vi "AlliGator Settings Event Refnum.vi"(1 "AlliGator Settings Event":T1, 3 "Error In":errorcluster) -> (7 "AlliGator Settings Event Refnum":refnum<user-event>, 9 "Error Out":errorcluster)   [LabVIEW 2021, in "AlliGator Settings.lvlib"]
doc: "Sends user event to the Settings window."
uses:
  AlliGator Settings.lvlib
  AlliGator Settings Event.ctl
  AlliGator Settings Window Messages.ctl
panel:
  # "see the AlliGator License on the block diagram (Ctrl+E or Window:Show Block Diagram)"
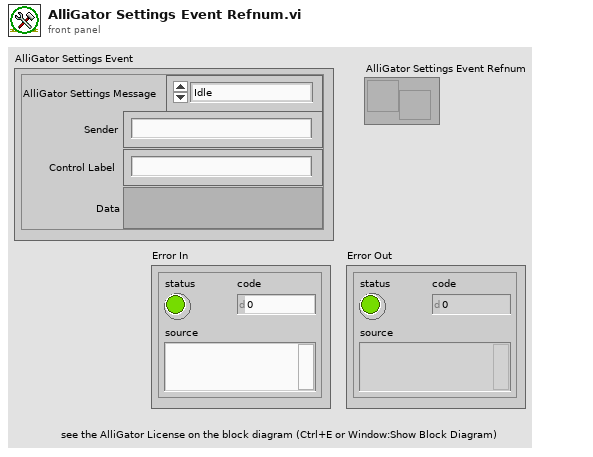
[diagram p1: front panel]
types:
  T1 = typedef "AlliGator Settings.lvlib/AlliGator Settings Event.ctl" = cluster{"AlliGator Settings Message":T2, "Sender":string, "Control Label":string, "Data":variant}
  T2 = typedef "AlliGator Settings.lvlib/AlliGator Settings Window Messages.ctl" = enum16{"Idle", "Subscribe", "Unsubscribe", "Refresh Parameter", "Refresh All Parameters", "Quit"}
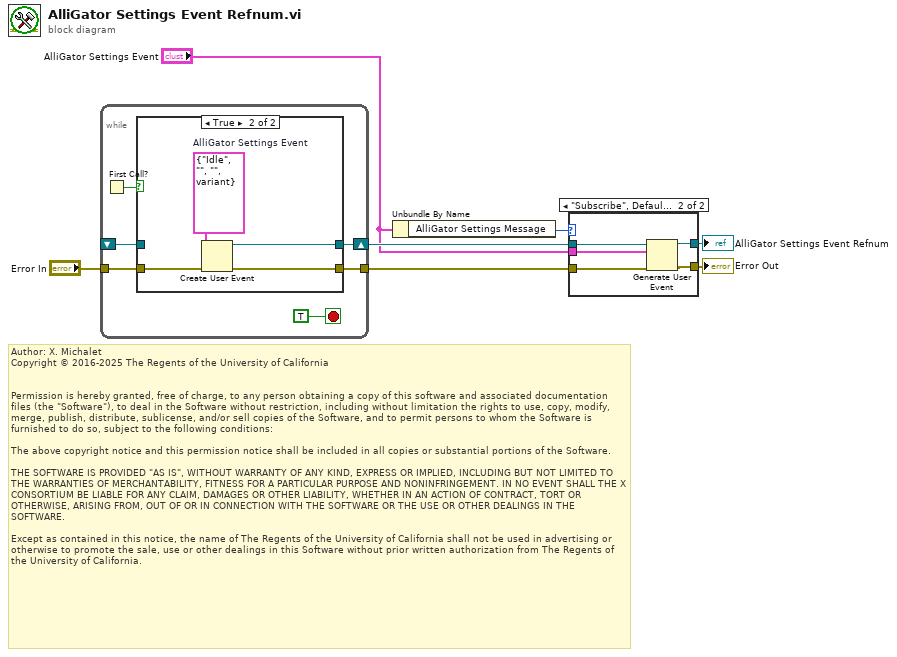
[diagram p0: block diagram]
diagram:
  # "Author: X. Michalet\nCopyright © 2016-2025 The Regents of the University of California\n \n\nPermission is hereby granted, free of charge, to any person obtaining a copy of this software and associated documentation files (the \"Software\"), to deal in the Software without restriction, including without limitation the rights to use, copy, modify, merge, publish, distribute, sublicense, and/or sell copies of the Software, and to permit persons to whom the Software is furnished to do so, subject to the following conditions:\n\nThe above copyright notice and this permission notice shall be included in all copies or substantial portions of the Software.\n\nTHE SOFTWARE IS PROVIDED \"AS IS\", WITHOUT WARRANTY OF ANY KIND, EXPRESS OR IMPLIED, INCLUDING BUT NOT LIMITED TO THE WARRANTIES OF MERCHANTABILITY, FITNESS FOR A PARTICULAR PURPOSE AND NONINFRINGEMENT. IN NO EVENT SHALL THE X CONSORTIUM BE LIABLE FOR ANY CLAIM, DAMAGES OR OTHER LIABILITY, WHETHER IN AN ACTION OF CONTRACT, TORT OR OTHERWISE, ARISING FROM, OUT OF OR IN CONNECTION WITH THE SOFTWARE OR THE USE OR OTHER DEALINGS IN THE SOFTWARE.\n\nExcept as contained in this notice, the name of The Regents of the University of California shall not be used in advertising or otherwise to promote the sale, use or other dealings in this Software without prior written authorization from The Regents of the University of California."
  n1 = while {
    shift-right: [w11] -> w5
    shift-left: _ -> [w10]
    tunnel: [w9] -> w6
    tunnel: "Error In" -> [w8]
    stop <- TRUE stop-if-true
    n2 = First Call?() -> (First Call?: T/F=w13:bool)
    n3 = case shown="True" w13 {
      tunnel: [w15 w19] -> w11
      tunnel: w10 -> [w15 _]
      tunnel: [w14 w18] -> w9
      tunnel: w8 -> [w14 w17]
      frame False {
      }
      frame True {
        w16 = T1 {"AlliGator Settings Message"=enum."Idle", "Sender"="", "Control Label"="", "Data"=variant}  # AlliGator Settings Event
        n4 = Create User Event(user event datatype=w16, error in=w17) -> (user event=w19:refnum<user-event>, error out=w18:errorcluster)
      }
    }
  }
  n5 = Unbundle By Name("AlliGator Settings Event") -> ("AlliGator Settings Message"=w1:T2)
  n6 = case shown="\"Subscribe\", Default" w1 {
    tunnel: w6 -> [w20 w26]
    tunnel: w5 -> [w21 w25]
    tunnel: [w20 w24] -> w4
    tunnel: "AlliGator Settings Event" -> [_ w23]
    tunnel: [w21 w22] -> w3
    frame "Idle" {
    }
    frame "Subscribe", Default {
      n7 = Generate User Event(user event=w25, event data cluster=w23, error in=w26) -> (user event out=w22:refnum<user-event>, error out=w24:errorcluster)  [unwired: 1 in]
    }
  }
  "Error Out" <- w4
  "AlliGator Settings Event Refnum" <- w3
